vi "Create Class.vi"(8 "error in (no error)":errorcluster, 10 "Y-Axis":refnum<class "iMotion Controller.lvclass">, 11 "X-Axis":refnum<class "iMotion Controller.lvclass">) -> (0 "error out":errorcluster, 3 "Sync 2-Axis Stage Controller out":refnum<class "Sync 2-Axis Stage Controller.lvclass">)   [LabVIEW 2022 SP3, in "Sync 2-Axis Stage Controller.lvclass"]
uses:
  Sync 2-Axis Stage Controller.lvclass
  Axis Objects/iMotion Controller/iMotion Controller.lvclass
  Sync 2-Axis Stage Controller.lvclass/Sync 2-Axis Stage Controller.ctl
  <vilib>/ErrorRing/Error Ring.xnode
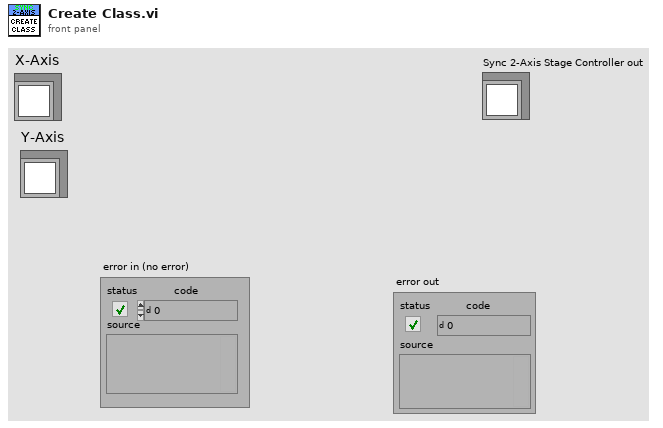
[diagram p1: front panel]
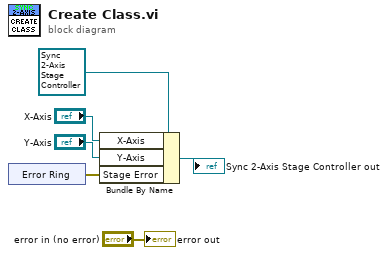
[diagram p0: block diagram]
diagram:
  n1 = xnode "Error Ring"() -> ("error out"=w1:errorcluster)
  n2 = Bundle By Name(cluster=refnum<class "Sync 2-Axis Stage Controller.lvclass"> refnum ("Sync 2-Axis Stage Controller in"), "X-Axis"="X-Axis", "Y-Axis"="Y-Axis", "Stage Error"=w1) -> (→"Sync 2-Axis Stage Controller out":refnum<class "Sync 2-Axis Stage Controller.lvclass">)
  "error out" <- "error in (no error)"
